vi "ProcessaSinalBaixa.vi"(0 "Sinais":waveform(dbl)[](array[waveform]), 2 "TxAmostragem":dbl=300.0 caption="Tx. Amostragem (Hz):" min=50.0 max=50000.0, 4 "TxAmostragemBaixa":dbl=300.0 caption="Tx. Baixa (Hz):" min=50.0 max=50000.0, 5 "Reset":bool) -> (14 "SinaisBaixa":waveform(dbl)[](array[waveform]))   [LabVIEW 2017]
uses:
  <vilib>/Analysis/3filter.llb/Filter Passband Type.ctl
  <vilib>/Analysis/3filter.llb/IIR Cascade Filter with I.C. (DBL).vi
  <vilib>/Analysis/2dsp.llb/Decimate (single shot, DBL).vi
  <vilib>/Analysis/NI_AALPro.lvlib
  <vilib>/Analysis/NI_AALBase.lvlib
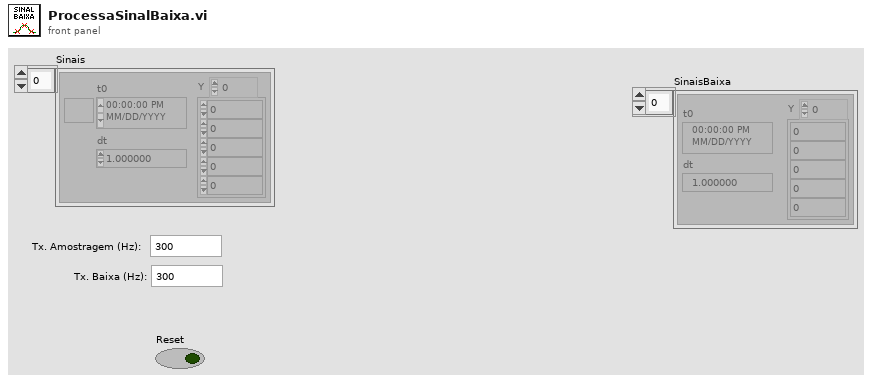
[diagram p1: front panel]
types:
  T1 = cluster{"filter structure":enum32{"IIR 2nd Order", "IIR 4th Order"}, "Reverse Coefficients":dbl[], "Forward Coefficients":dbl[]}
  T2 = typedef "NI_AALBase.lvlib/Filter Passband Type.ctl" = enum32{"Lowpass", "Highpass", "Bandpass", "Bandstop"}
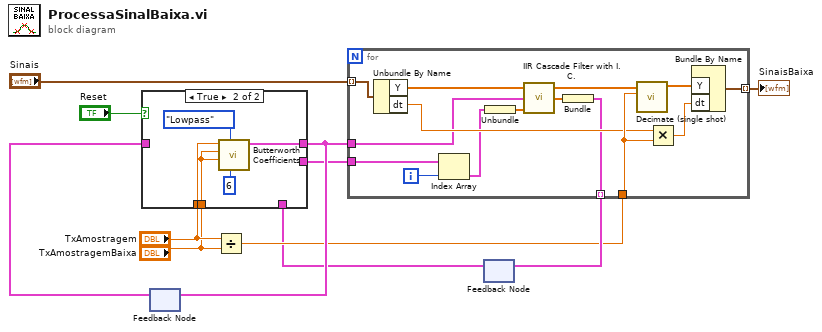
[diagram p0: block diagram]
diagram:
  n1 = feedback #1() -> (w11:T1)  [unwired: 1 in]
  n2 = Divide(x="TxAmostragem", y="TxAmostragemBaixa") -> (x/y=w8:dbl)
  n3 = feedback #2() -> (w4:cluster{"Final Filter State":dbl[]}[])  [unwired: 1 in]
  n4 = case shown="True" "Reset" {
    tunnel: "TxAmostragem" -> [_ w18]
    tunnel: "TxAmostragemBaixa" -> [_ w17]
    tunnel: [w13 w14] -> w10
    tunnel: w11 -> [w13 _]
    tunnel: [w12 _] -> w5
    tunnel: w4 -> [w12 _]
    frame False {
    }
    frame True {
      n5 = call <vilib>:"Butterworth Coefficients.vi"("order"=6, "filter type"=Filter_Passband_Type."Lowpass", "low cutoff freq: fl"=w17, "high cutoff freq: fh"=w17, "sampling freq: fs"=w18) -> ("IIR Filter Cluster"=w14:T1)  [unwired: 5 in, 1 out]
    }
  }
  n6 = feedback-in #1(w10) -> ()
  n7 = for {
    tunnel: w8 -> [w32]
    tunnel: [w30] -> w7 mode=indexing
    tunnel: "Sinais" -> [w29] mode=indexing
    tunnel: w10 -> [w26]
    tunnel: [w21] -> w9 mode=indexing
    tunnel: w5 -> [w19]
    i -> [w23]
    n8 = Unbundle By Name(w29) -> ("Y"=w28:dbl[], "dt"=w27:dbl)
    n9 = Index Array(array=w19, index=w23) -> (element=w22:cluster{"Final Filter State":dbl[]})
    n10 = Unbundle(w22) -> ("Final Filter State"=w20:dbl[])
    n11 = call-poly <vilib>:"IIR Cascade Filter with I.C..vi"("Initial Filter State"=w20, "IIR Filter Cluster"=w26, "X"=w28) -> ("Final Filter State"=w24:dbl[], "Filtered X"=w25:dbl[])  [unwired: 1 out]
    n12 = Bundle("Final Filter State"=w24) -> (w21:cluster{"Final Filter State":dbl[]})  [unwired: 1 in]
    n13 = call-poly <vilib>:"Decimate (single shot).vi"("decimating factor"=w32, "X"=w25) -> ("Decimated Array"=w33:dbl[])  [unwired: 8 in, 1 out]
    n14 = Multiply(x=w27, y=w32) -> (x*y=w31:dbl)
    n15 = Bundle By Name("Y"=w33, "dt"=w31) -> (w30:waveform(dbl))  [unwired: 1 in]
  }
  "SinaisBaixa" <- w7
  n16 = feedback-in #2(w9) -> ()
